vi "setImplicitParameterNode.vi"(0 "reference":refnum<class "CallNode.lvclass">, 1 "objectCallNodeRef":refnum<class "AbstractNode.lvclass">, 5 "error in (no error)":errorcluster) -> (14 "reference out":refnum<class "CallNode.lvclass">, 19 "error out":errorcluster)   [LabVIEW 2016, in "CallNode.lvclass"]
uses:
  <resource>/Framework/Providers/Open_GDS/UML/CallNode_class/CallNode.lvclass
  <resource>/Framework/Providers/Open_GDS/UML/AbstractNode_class/AbstractNode.lvclass
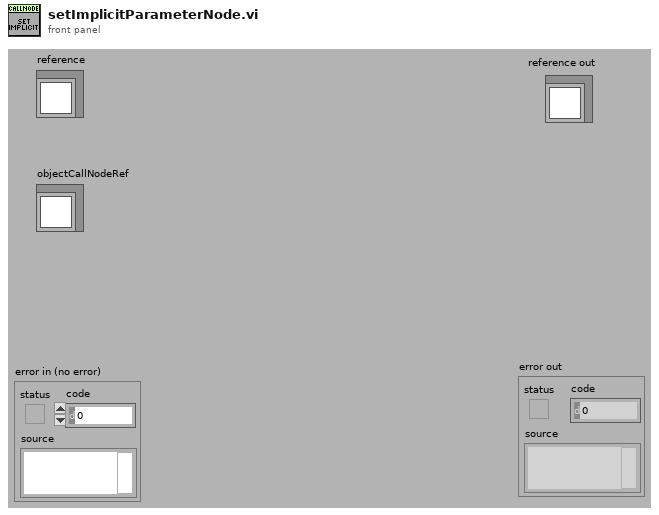
[diagram p1: front panel]
types:
  T1 = typedef "CallNode.lvclass/ObjectAttributes.ctl" = cluster{"objectCallNodeRef":refnum<class "AbstractNode.lvclass">, "signaled":bool, "openBottom":bool, "DEFAULT_WIDTH":i32, "DEFAULT_HEIGHT":i32, "CALL_YGAP":i32}
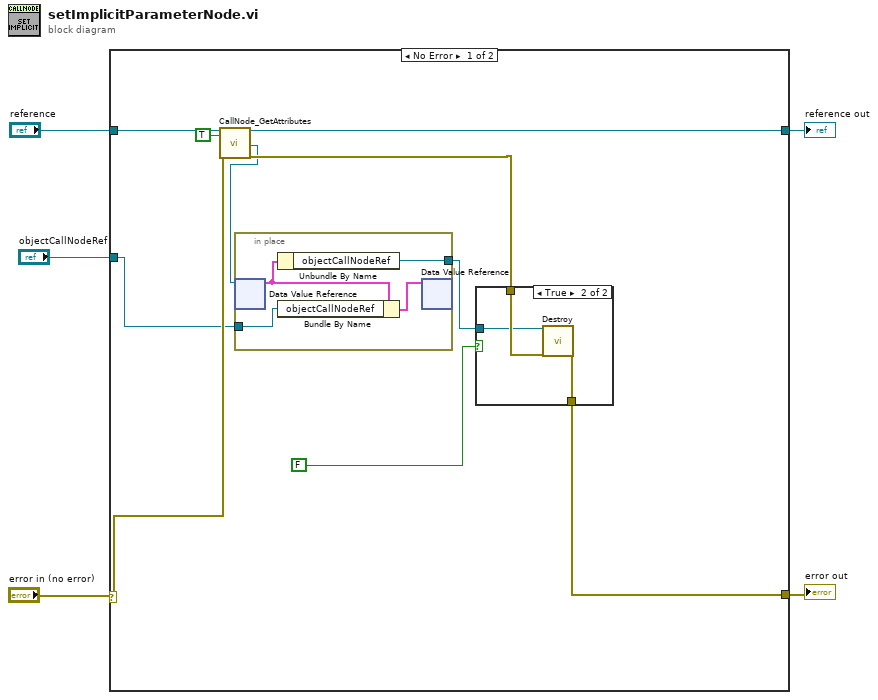
[diagram p0: block diagram]
diagram:
  n1 = case shown="No Error" "error in (no error)" {
    selector: "error in (no error)" -> [w12 w24]
    tunnel: "reference" -> [w15 w25]
    tunnel: [w14 w24] -> w4
    tunnel: [w13 w25] -> w3
    tunnel: "objectCallNodeRef" -> [w6 _]
    frame No Error {
      n2 = call <resource>:"CallNode_GetAttributes.vi"("reference in"=w15, "OnlyGetDvrReference(False)"=TRUE, "error in (no error)"=w12) -> ("reference out"=w13:refnum<class "CallNode.lvclass">, "DataRef"=w8:refnum<data-value>, "error out"=w11:errorcluster)  [unwired: 13 in, 1 out]
      n3 = in-place {
        in-place-border: [w18] -> w7
        in-place-border: w6 -> [w17]
        n4 = in-place-dvr #1(w8) -> (w19:T1)  [unwired: 1 out]
        n5 = Unbundle By Name(w19) -> ("objectCallNodeRef"=w18:refnum<class "AbstractNode.lvclass">)
        n6 = Bundle By Name(cluster=w19, "objectCallNodeRef"=w17) -> (w16:T1)
        n7 = in-place-dvr #1(w16) -> ()  [unwired: 2 out]
      }
      n8 = case shown="True" FALSE ("Case Constant\n(See Context Help)") {
        tunnel: w7 -> [_ w21]
        tunnel: w11 -> [w20 w23]
        tunnel: [w20 w22] -> w14
        frame False {
        }
        frame True {
          n9 = call-dynamic "Destroy.vi"("reference"=w21, "error in (no error)"=w23) -> ("error out"=w22:errorcluster)  [unwired: 16 in, 1 out]
        }
      }
    }
    frame Error {
    }
  }
  "reference out" <- w3
  "error out" <- w4
